vi "Score.vi"(6 "Max Depth (8)":i32=7, 8 "Depth":i32, 10 "SpielerZuege":i32, 11 "Game":i32[][](array[numeric])) -> (1 "Game over":bool, 2 "Win":bool, 3 "Score":i32)   [LabVIEW 2017]
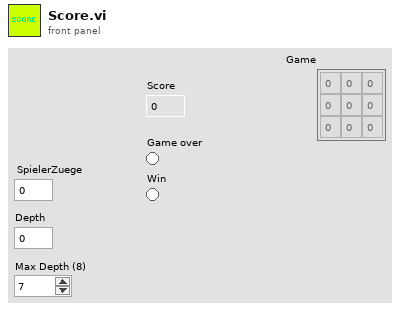
[diagram p1: front panel]
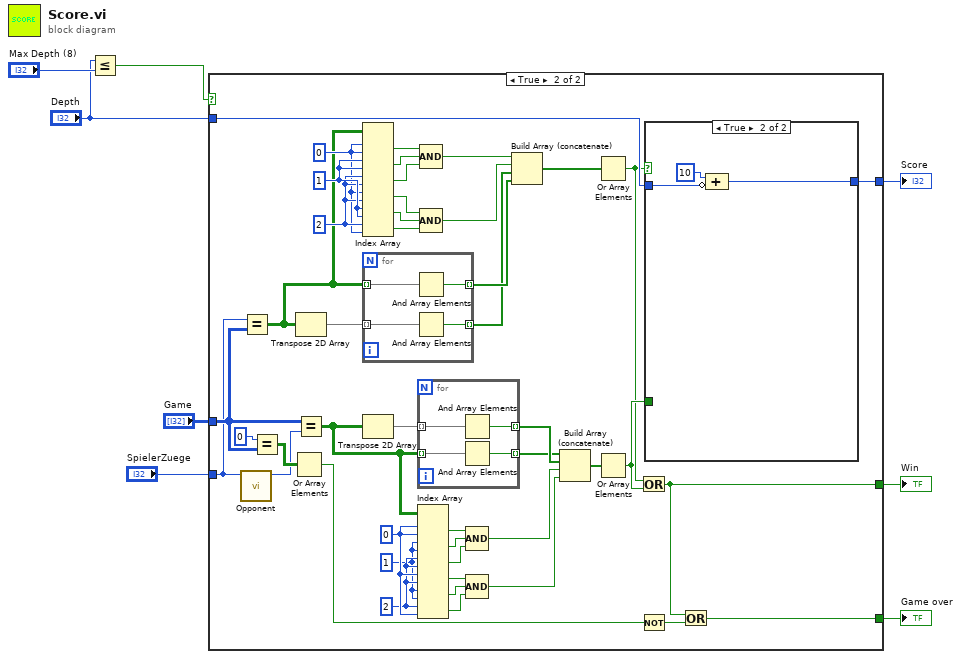
[diagram p0: block diagram]
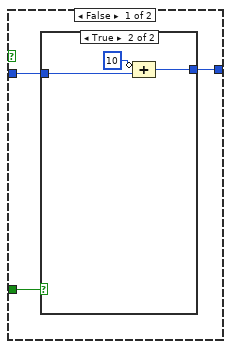
[diagram p3: hidden frame]
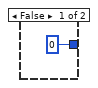
[diagram p4: hidden frame]
diagram:
  n1 = Less Or Equal?(x="Depth", y="Max Depth (8)") -> (x <= y?=w2:bool)
  n2 = case shown="True" w2 {
    tunnel: [_ w40] -> w8
    tunnel: [_ w35] -> w7
    tunnel: "Game" -> [_ w18]
    tunnel: "SpielerZuege" -> [_ w17]
    tunnel: "Depth" -> [_ w41]
    tunnel: [_ w10] -> w1
    frame False {
    }
    frame True {
      w25 = 2 ("index (row)")
      w24 = 1 ("index (row)")
      w26 = 0 ("index (row)")
      w49 = 2 ("index (row)")
      w50 = 1 ("index (row)")
      w48 = 0 ("index (row)")
      n3 = call "Opponent.vi"("Player"=w17) -> ("Opponent"=w16:i32)  [unwired: 10 in]
      n4 = Equal?(x=w17, y=w18) -> (x = y?=w9:bool[][])
      n5 = Equal?(x=0 ("index (row)"), y=w18) -> (x = y?=w38:bool[][])
      n6 = Or Array Elements(Boolean array=w38) -> (logical OR=w37:bool)
      n7 = Transpose 2D Array(2D array=w9) -> (transposed array=w53:bool[][])
      n8 = Equal?(x=w18, y=w16) -> (x = y?=w23:bool[][])
      n9 = Index Array(array=w9, index (row) #1=w48, index (col) #1=w48, index (row) #2=w50, index (col) #2=w50, index (row) #3=w49, index (col) #3=w49, index (row) #4=w48, index (col) #4=w49, index (row) #5=w50, index (col) #5=w50, index (row) #6=w49, index (col) #6=w48) -> (element #1=w47:bool, element #2=w46:bool, element #3=w45:bool, element #4=w43:bool, element #5=w44:bool, element #6=w42:bool)
      n10 = for {
        tunnel: w9 -> [w71] mode=indexing
        tunnel: w53 -> [w70] mode=indexing
        tunnel: [w69] -> w15 mode=indexing
        tunnel: [w68] -> w52 mode=indexing
        n11 = And Array Elements(Boolean array=w71) -> (logical AND=w68:bool)
        n12 = And Array Elements(Boolean array=w70) -> (logical AND=w69:bool)
      }
      n13 = Transpose 2D Array(2D array=w23) -> (transposed array=w19:bool[][])
      n14 = for {
        tunnel: w23 -> [w57] mode=indexing
        tunnel: w19 -> [w56] mode=indexing
        tunnel: [w55] -> w22 mode=indexing
        tunnel: [w54] -> w20 mode=indexing
        n15 = And Array Elements(Boolean array=w56) -> (logical AND=w55:bool)
        n16 = And Array Elements(Boolean array=w57) -> (logical AND=w54:bool)
      }
      n17 = Index Array(array=w23, index (row) #1=w26, index (col) #1=w26, index (row) #2=w24, index (col) #2=w24, index (row) #3=w25, index (col) #3=w25, index (row) #4=w26, index (col) #4=w25, index (row) #5=w24, index (col) #5=w24, index (row) #6=w25, index (col) #6=w26) -> (element #1=w27:bool, element #2=w28:bool, element #3=w29:bool, element #4=w31:bool, element #5=w30:bool, element #6=w32:bool)
      n18 = Compound Arithmetic op=AND(w47, w46, w45) -> (w13:bool)
      n19 = Compound Arithmetic op=AND(w43, w44, w42) -> (w14:bool)
      n20 = Compound Arithmetic op=AND(w27, w28, w29) -> (w33:bool)
      n21 = Compound Arithmetic op=AND(w31, w30, w32) -> (w34:bool)
      n22 = Build Array (concatenate)(w13, w14, w15, w52) -> (w51:bool[])
      n23 = Build Array (concatenate)(w20, w22, w33, w34) -> (w21:bool[])
      n24 = Or Array Elements(Boolean array=w51) -> (logical OR=w11:bool)
      n25 = Or Array Elements(Boolean array=w21) -> (logical OR=w12:bool)
      n26 = Or(x=w11, y=w12) -> (x .or. y?=w10:bool)
      n27 = Not(x=w37) -> (.not. x?=w36:bool)
      n28 = case shown="True" w11 {
        tunnel: w41 -> [w60 w67]
        tunnel: [w59 w65] -> w40
        tunnel: w12 -> [w58 _]
        frame False {
          n29 = case shown="True" w58 {
            tunnel: w60 -> [_ w64]
            tunnel: [0 w62] -> w59
            frame False {
            }
            frame True {
              n30 = Compound Arithmetic op=ADD(invert 10 ("x"), w64) -> (w62:i32)
            }
          }
        }
        frame True {
          n31 = Compound Arithmetic op=ADD(10 ("x"), invert w67) -> (w65:i32)
        }
      }
      n32 = Or(x=w10, y=w36) -> (x .or. y?=w35:bool)
    }
  }
  "Score" <- w8
  "Game over" <- w7
  "Win" <- w1
